vi "Memory Define Location Name.vi"(7 "error in (no error)":errorcluster, 8 "Name":string, 9 "Memory Location":u32=1 min=1 max=99 step=1, 10 "VISA resource name":refnum<visa-resource-name>) -> (0 "error out":errorcluster, 3 "VISA resource name out":refnum<visa-resource-name>)   [LabVIEW 2025, in "Chroma 19052.lvlib"]
doc: "Contact Chroma\nTEL: +886-2-2298-3855 \nTEL: +886-3-397-5788 \nFAX: +886-2-2298-3596\nFAX: +886-3-327-4703 \nURL: http://www.chromaate.com \nE-mail: chroma@chroma.com.tw"
uses:
  <instrlib>/Chroma 19052/Chroma 19052.lvlib
panel:
  # "1...99"
  # "Define Location Name only\nWARNING: Does not save instrument configuration"
  # "allowed characters: 0~9, A~Z, -"
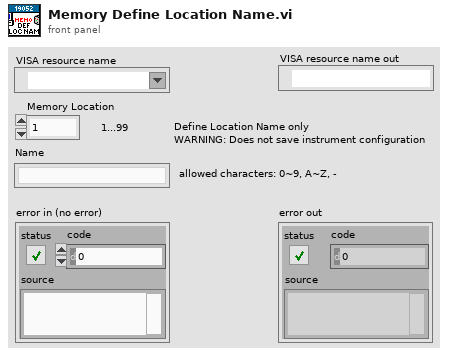
[diagram p1: front panel]
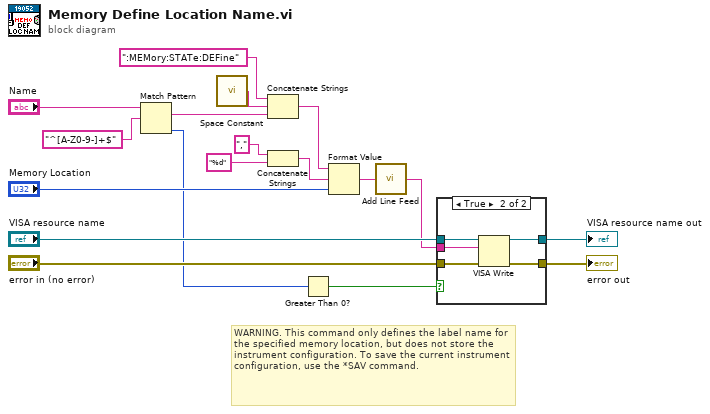
[diagram p0: block diagram]
diagram:
  # "WARNING. This command only defines the label name for the specified memory location, but does not store the instrument configuration. To save the current instrument configuration, use the *SAV command."
  n1 = Match Pattern(string="Name", regular expression="^[A-Z0-9-]+$") -> (match substring=w2:string, offset past match=w5:i32)  [unwired: 1 in, 2 out]
  n2 = call <vilib>:"Space Constant.vi"() -> ("String"=w9:string)
  n3 = Concatenate Strings(":MEMory:STATe:DEFine", w9, w2) -> (w18:string)
  n4 = Concatenate Strings("," ("string"), "%d") -> (w6:string)
  n5 = Greater Than 0?(x=w5) -> (x > 0?=w1:bool)
  n6 = Format Value(string ("")=w18, format string=w6, value (0)="Memory Location") -> (output string=w17:string)
  n7 = call <instrlib>:"Add Line Feed.vi"("Command string"=w17) -> ("Concatenated string"=w11:string)  [unwired: 4 in]
  n8 = case shown="True" w1 {
    tunnel: "error in (no error)" -> [w20 w25]
    tunnel: "VISA resource name" -> [w19 w24]
    tunnel: [w20 w23] -> w13
    tunnel: [w19 w22] -> w12
    tunnel: w11 -> [_ w21]
    frame False {
    }
    frame True {
      n9 = VISA Write(VISA resource name=w24, write buffer=w21, error in (no error)=w25) -> (VISA resource name out=w22:refnum<visa-resource-name>, error out=w23:errorcluster)  [unwired: 1 out]
    }
  }
  "error out" <- w13
  "VISA resource name out" <- w12
